vi "Crop.vi"(0 "image in":refnum<class "MSC Image.lvclass">, 1 "Bounding Box":T1, 5 "error in (no error)":errorcluster) -> (14 "image out":refnum<class "MSC Image.lvclass">, 15 "Coerced Bounding Box":T1, 19 "error out":errorcluster)   [LabVIEW 2014, in "MSC Image.lvclass"]
doc: "Crops the image to the selected size."
uses:
  MSC Image.lvclass
  controls/Contour.ctl
  MSC Image.lvclass/MSC Image.ctl
  Dependencies/x86/MSC I Process32.dll
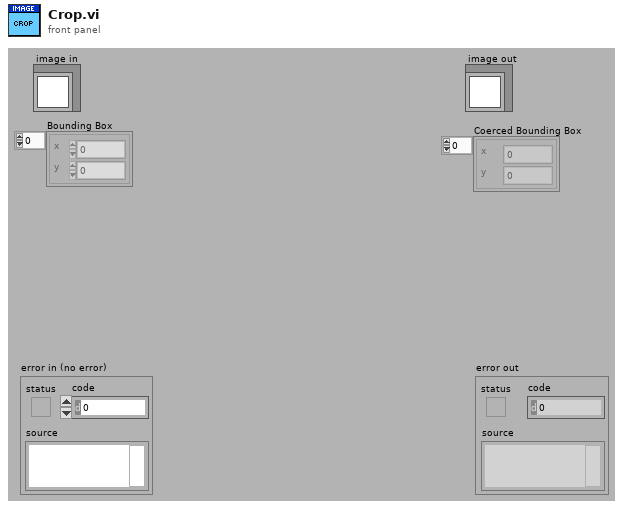
[diagram p1: front panel]
types:
  T1 = typedef "MSC Image.lvclass/Contour.ctl" = cluster{"x":i16, "y":i16}[]
  T2 = typedef "MSC Image.lvclass/Size.ctl" = cluster{"Cols":i32, "Rows":i32}
  T3 = typedef "Image.ctl" = cluster{"Pointer":u64, "Size":T4, "Image Type":T5, "Time Stamp":timestamp, "Variant":variant}
  T4 = typedef "Size.ctl" = cluster{"Cols":i32, "Rows":i32}
  T5 = typedef "Image Type.ctl" = i32
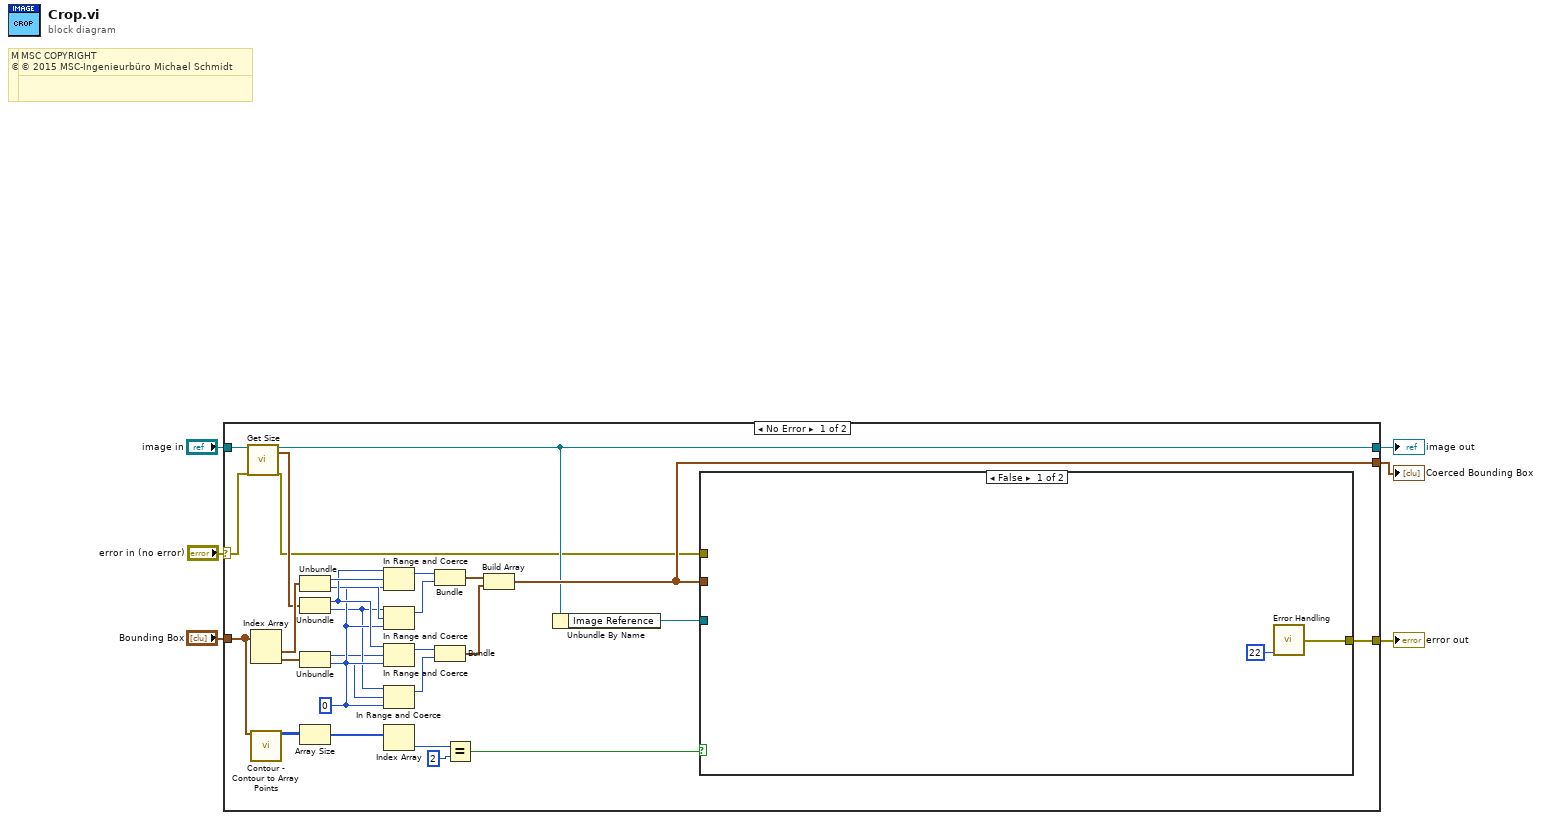
[diagram p0: block diagram]
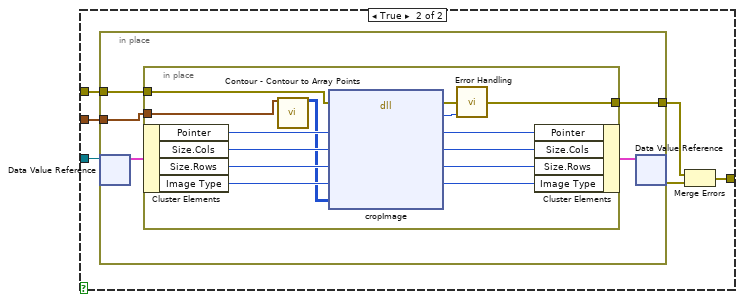
[diagram p2: hidden frame]
diagram:
  # "MSC COPYRIGHT\n© 2016 MSC-Ingenieurbüro Michael Schmidt"
  # "MSC COPYRIGHT\n© 2016 MSC-Ingenieurbüro Michael Schmidt"
  # "MSC COPYRIGHT\n© 2015 MSC-Ingenieurbüro Michael Schmidt"
  # "MSC COPYRIGHT\n© 2015 MSC-Ingenieurbüro Michael Schmidt"
  n1 = case shown="No Error" "error in (no error)" {
    selector: "error in (no error)" -> [w8 w64]
    tunnel: [w35 w64] -> w1
    tunnel: [w10 w63] -> w6
    tunnel: "image in" -> [w12 w63]
    tunnel: "Bounding Box" -> [w29 _]
    tunnel: [w15 _] -> w3
    frame No Error {
      w23 = i16 0 ("lower limit")
      n2 = call-dynamic "Get Size.vi"("image in"=w12, "error in (no error)"=w8) -> ("image out"=w10:refnum<class "MSC Image.lvclass">, "Size"=w11:T2, "error out"=w7:errorcluster)  [unwired: 15 in]
      n3 = Index Array(array=w29) -> (element #1=w28:cluster{"x":i16, "y":i16}, element #2=w27:cluster{"x":i16, "y":i16})  [unwired: 2 in]
      n4 = call "Contour - Contour to Array Points.vi"("Contour"=w29) -> ("Array Points"=w30:i16[][])  [unwired: 14 in]
      n5 = Unbundle(w28) -> ("x"=w26:i16, "y"=w24:i16)
      n6 = Unbundle(w11) -> ("Cols"=w25:i32, "Rows"=w22:i32)
      n7 = Unbundle(w27) -> ("x"=w14:i16, "y"=w13:i16)
      n8 = Array Size(array=w30) -> (size(s)=w34:i32[])
      n9 = In Range and Coerce(upper limit=w25, x=w26, lower limit=w23) -> (coerced(x)=w21:i32)  [unwired: 1 out]
      n10 = In Range and Coerce(upper limit=w22, x=w24, lower limit=w23) -> (coerced(x)=w19:i32)  [unwired: 1 out]
      n11 = In Range and Coerce(upper limit=w25, x=w14, lower limit=w23) -> (coerced(x)=w20:i32)  [unwired: 1 out]
      n12 = In Range and Coerce(upper limit=w22, x=w13, lower limit=w23) -> (coerced(x)=w18:i32)  [unwired: 1 out]
      n13 = Index Array(array=w34) -> (element=w33:i32)  [unwired: 1 in]
      n14 = Bundle("Cols"=w21, "Rows"=w19) -> (w17:cluster{"Cols":i32, "Rows":i32})  [unwired: 1 in]
      n15 = Bundle("Cols"=w20, "Rows"=w18) -> (w16:cluster{"Cols":i32, "Rows":i32})  [unwired: 1 in]
      n16 = Equal?(x=w33, y=2) -> (x = y?=w31:bool)
      n17 = Build Array(w17, w16) -> (w15:cluster{"Cols":i32, "Rows":i32}[])
      n18 = Unbundle By Name(w10) -> ("Image Reference"=w9:refnum<data-value>)
      n19 = case shown="False" w31 {
        tunnel: w7 -> [_ w41]
        tunnel: w9 -> [_ w40]
        tunnel: [w36 w39] -> w35
        tunnel: w15 -> [_ w38]
        frame False {
          n20 = call "Error Handling.vi"("return type"=22) -> ("error out"=w36:errorcluster)  [unwired: 13 in, 1 out]
        }
        frame True {
          n21 = in-place {
            in-place-border: w41 -> [w46]
            in-place-border: [w45] -> w42
            in-place-border: w38 -> [w44]
            n22 = in-place-dvr #1(w40) -> (w47:T3)  [unwired: 1 out]
            n23 = in-place {
              in-place-border: w46 -> [w57]
              in-place-border: [w62] -> w45
              in-place-border: w44 -> [w50]
              n24 = in-place-cluster #2(w47) -> ("Pointer"=w61:u64, "Size.Cols"=w52:i32, "Size.Rows"=w51:i32, "Image Type"=w54:T5)
              n25 = call "Contour - Contour to Array Points.vi"("Contour"=w50) -> ("Array Points"=w49:i16[][])  [unwired: 14 in]
              n26 = dll-call lib="C:/Users/MSC/LabVIEW Projekte/LV 2014/MSC I-Process/user.lib/MSC-I Process/Dependencies/x86/MSC I Process*.dll" fn="cropImage"(error in=w57, "pointer"=w61, "cols"=w52, "rows"=w51, "type"=w54, "boundingBoxPoints"=w49) -> (error out=w56:errorcluster, "error"=w55:i32, "pointer"=w60:u64, "cols"=w59:i32, "rows"=w58:i32, "type"=w53:i32)  [unwired: 3 in, 1 out]
              n27 = call "Error Handling.vi"("error in (no error)"=w56, "return type"=w55) -> ("error out"=w62:errorcluster)  [unwired: 12 in, 1 out]
              n28 = in-place-cluster #2("Pointer"=w60, "Size.Cols"=w59, "Size.Rows"=w58, "Image Type"=w53) -> (w48:T3)
            }
            n29 = in-place-dvr #1(w48) -> (w43:errorcluster)  [unwired: 1 out]
          }
          n30 = Merge Errors(w42, w43) -> (w39:errorcluster)
        }
      }
    }
    frame Error {
    }
  }
  "error out" <- w1
  "image out" <- w6
  "Coerced Bounding Box" <- w3
